vi "SCI_Tx_Index_0x01.vi"(1 "输入数据包（簇）":T1 {"包头" format="%02x"; "数据低8位" format="%02x"; "数据低高8位" format="%02x"; "数据类型" items=["VOID"]; "CRC余数" format="%02x"}, 2 "下一包数据（簇）":T1={"包头"=170, "数据低8位"=0, "数据低高8位"=0, "数据类型"=0, "CRC余数"=0, "数据无效"=FALSE, "数据更新"=FALSE} {"包头" format="%02x"; "数据低8位" format="%02x"; "数据低高8位" format="%02x"; "数据类型" items=["VOID"]; "CRC余数" format="%02x"}) -> (6 "上一个包数据（簇）":T1={"包头"=170, "数据低8位"=0, "数据低高8位"=0, "数据类型"=0, "CRC余数"=0, "数据无效"=FALSE, "数据更新"=FALSE} {"包头" format="%02x"; "数据低8位" format="%02x"; "数据低高8位" format="%02x"; "数据类型" items=["VOID"]; "CRC余数" format="%02x"})   [LabVIEW 2015]
uses:
  SCI_DataPck.ctl
  SCI_DataType.ctl
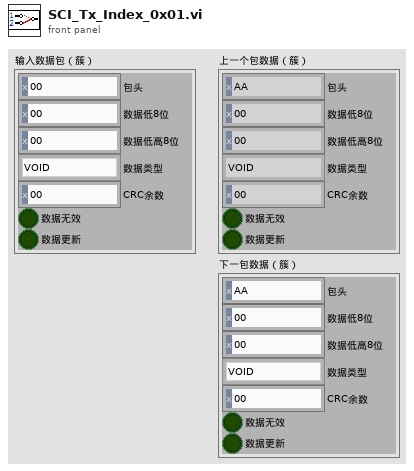
[diagram p1: front panel]
types:
  T1 = typedef "SCI_DataPck.ctl" = cluster{"包头":u16, "数据低8位":u16, "数据低高8位":u16, "数据类型":T2, "CRC余数":u16, "数据无效":bool, "数据更新":bool}
  T2 = typedef "SCI_DataType.ctl" = u16
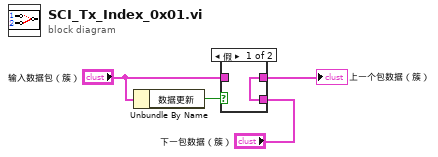
[diagram p0: block diagram]
diagram:
  n1 = Unbundle By Name("输入数据包（簇）") -> ("数据更新"=w3:bool)
  n2 = case shown="假" w3 {
    tunnel: [w5 w6] -> w2
    tunnel: "输入数据包（簇）" -> [_ w6]
    tunnel: "下一包数据（簇）" -> [w5 _]
    frame False {
    }
    frame True {
    }
  }
  "上一个包数据（簇）" <- w2
